vi "Zero window.vi"(6 "last adress":u32, 7 "First adress":u32, 8 "input valid":bool=TRUE, 10 "Address":u32, 11 "Value in":fxp<+/-,32,14>) -> (0 "output valid":bool=TRUE, 2 "Address out":u32, 3 "Value out":fxp<+/-,32,14>)   [LabVIEW 2018]
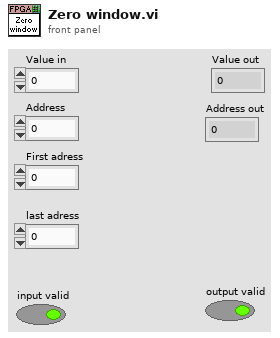
[diagram p1: front panel]
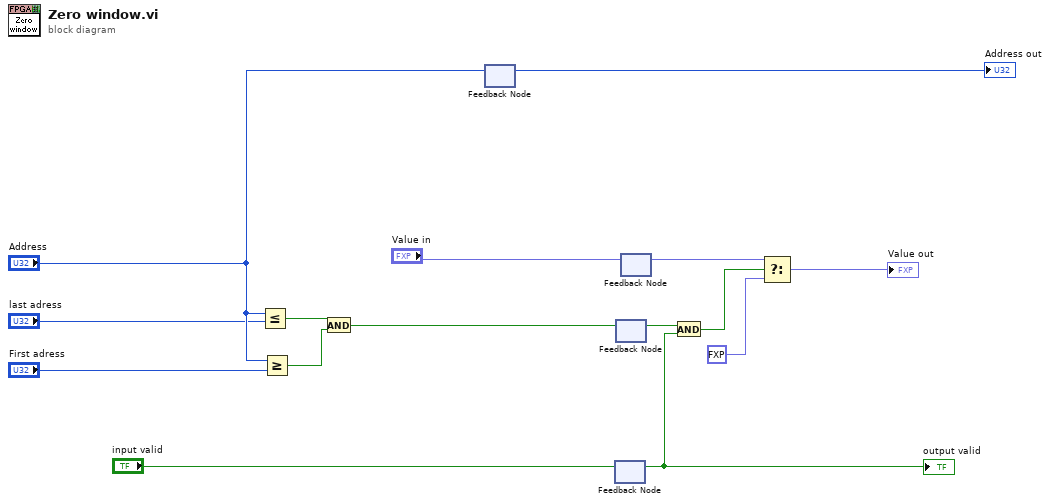
[diagram p0: block diagram]
diagram:
  n1 = Less Or Equal?(x="Address", y="last adress") -> (x <= y?=w10:bool)
  n2 = Greater Or Equal?(x="Address", y="First adress") -> (x >= y?=w9:bool)
  n3 = And(x=w10, y=w9) -> (x .and. y?=w8:bool)
  n4 = feedback #1() -> (→"Address out":u32)  [unwired: 1 in]
  n5 = feedback-in #1("Address") -> ()
  n6 = feedback #2() -> (w2:bool)  [unwired: 1 in]
  "output valid" <- w2
  n7 = feedback-in #2("input valid") -> ()
  n8 = feedback #3() -> (w5:bool)  [unwired: 1 in]
  n9 = feedback-in #3(w8) -> ()
  n10 = feedback-in #4("Value in") -> ()
  n11 = feedback #4() -> (w14:fxp<+/-,32,14>)  [unwired: 1 in]
  n12 = And(x=w5, y=w2) -> (x .and. y?=w4:bool)
  n13 = Select(t=w14, s=w4, f=fxp<+/-,32,14> 0.0) -> (s? t:f=→"Value out":fxp<+/-,32,14>)
